vi "Modular Test.vi"() -> ()   [LabVIEW 2018]
uses:
  Classes/Realsense Cam/Private/Stream Config STYP.ctl
  Classes/Realsense Cam/Private/Stream Types Enum STYP.ctl
  Classes/Message/Message.lvclass
  Classes/Video Cam Processor/Video Cam Processor.lvclass
  C:/Users/aaron.jencks/Documents/GitHub/emerson_seed_object_detection/LabVIEW/Projects/Paul's Video Viewer/Classes/Realsense Cam Video File Wrapper/Realsense Cam File Wrapper.lvclass
  C:/Users/aaron.jencks/Documents/GitHub/emerson_seed_object_detection/LabVIEW/Projects/Paul's Video Viewer/Classes/Video Processor/Video Processor.lvclass
  Classes/Frame Data Message/Frame Data Message.lvclass
  C:/Users/aaron.jencks/Documents/GitHub/emerson_seed_object_detection/LabVIEW/Projects/Paul's Video Viewer/Classes/Message/Message.lvclass
  Classes/STOP Message/STOP.lvclass
  Classes/Realsense Cam/Realsense Cam.lvclass
  Classes/Image Processing Handler/Image Processing Handler.lvclass
panel:
  out "Image":T1(plugin-control)
  in  "stop":bool
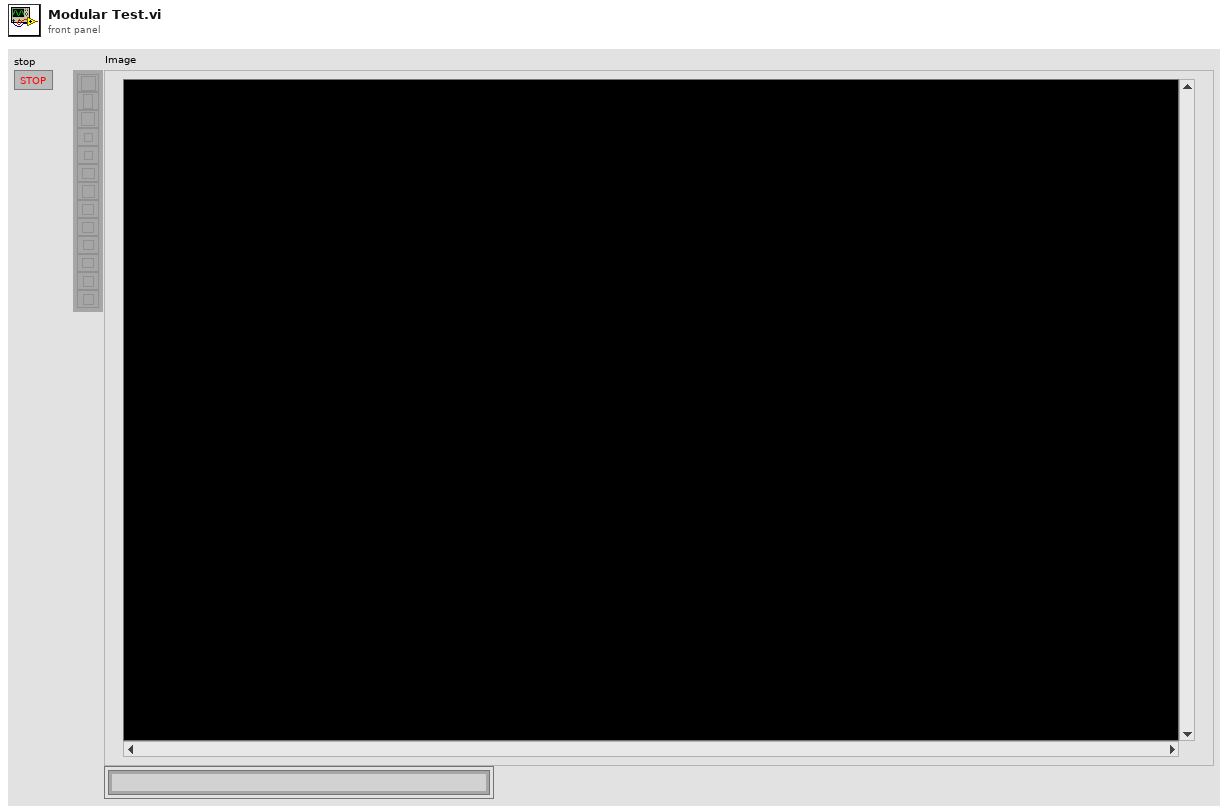
[diagram p1: front panel]
types:
  T1 = typedef "IMAQ Image.ctl" = refnum<image>
  T2 = typedef "Realsense Cam.lvclass/Stream Config STYP.ctl" = cluster{"Stream Type":T3, "Resolution":u16}
  T3 = typedef "Realsense Cam.lvclass/Stream Types Enum STYP.ctl" = enum16{"Depth", "Left IR", "Left IR Unrectified", "Right IR", "Right IR Unrectified", "Color", "RGB Ext."}
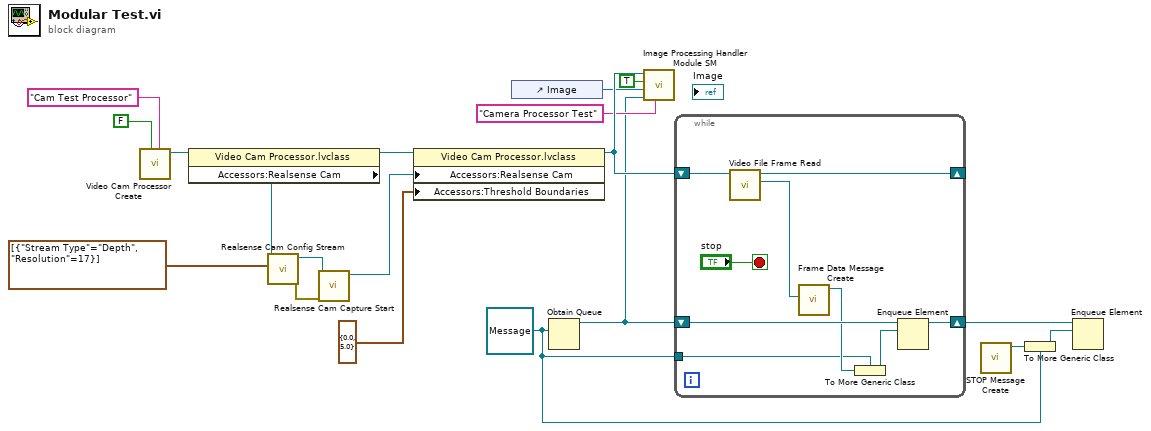
[diagram p0: block diagram]
diagram:
  w2 = refnum<class "Message.lvclass"> refnum ("Message.lvclass")
  n1 = call "Video Cam Processor Create.vi"("Identifier"="Cam Test Processor", "Open? (T)"=FALSE) -> ("Video Processor out"=w16:refnum<class "Video Cam Processor.lvclass">)  [unwired: 8 in, 1 out]
  n2 = property class="Video Cam Processor.lvclass"(reference=w16) -> (reference out=w13:refnum<class "Video Cam Processor.lvclass">, "Accessors:Realsense Cam"=w15:refnum<class "Realsense Cam.lvclass">)  [unwired: 1 in, 1 out]
  n3 = call-dynamic "Realsense Cam Config Stream.vi"("Streams"=T2[] [{"Stream Type"=enum."Depth", "Resolution"=17}], "Realsense Cam in"=w15) -> ("error out"=w17:errorcluster, "Realsense Cam out"=w18:refnum<class "Realsense Cam.lvclass">)  [unwired: 8 in]
  n4 = call-dynamic "Realsense Cam Capture Start.vi"("error in (no error)"=w17, "Realsense Cam in"=w18) -> ("Realsense Cam out"=w12:refnum<class "Realsense Cam.lvclass">)  [unwired: 7 in, 2 out]
  n5 = property class="Video Cam Processor.lvclass"(reference=w13, "Accessors:Realsense Cam"=w12, "Accessors:Threshold Boundaries"=cluster{"Minimum":dbl, "Maximum":dbl} {"Minimum"=0.0, "Maximum"=5.0} ("Threshold Boundaries")) -> (reference out=w9:refnum<class "Video Cam Processor.lvclass">)  [unwired: 1 in, 1 out]
  n6 = control-ref of="Image"() -> (w7:refnum<vi>)
  n7 = Obtain Queue(element data type=w2) -> (queue out=w5:refnum<queue>)  [unwired: 4 in, 2 out]
  n8 = call "Image Processing Handler Module SM.vi"("Identifier"="Camera Processor Test", "data queue"=w5, "Image Ctl Refnum"=w7, "Camera? (F)"=TRUE, "Video Processor"=w9) -> ()  [unwired: 7 in]
  n9 = while {
    shift-right: [w21] -> _
    shift-left: w9 -> [w28]
    tunnel: w2 -> [w23]
    shift-right: [w20] -> w4
    shift-left: w5 -> [w25]
    stop <- "stop" stop-if-true
    n10 = call-dynamic "Video File Frame Read.vi"("Video Processor in"=w28) -> ("Video Frame out"=w26:refnum<class "Video Frame.lvclass">, "Video Processor out"=w21:refnum<class "Video Cam Processor.lvclass">)  [unwired: 6 in, 3 out]
    n11 = call "Frame Data Message Create.vi"("Video Frame"=w26) -> ("Frame Data Message out"=w24:refnum<class "Frame Data Message.lvclass">)  [unwired: 9 in, 1 out]
    n12 = To More Generic Class(target class=w23, reference=w24) -> (generic class reference=w22:refnum<class "Message.lvclass">)
    n13 = Enqueue Element(queue=w25, element=w22) -> (queue out=w20:refnum<queue>)  [unwired: 2 in, 2 out]
  }
  n14 = call "STOP Message Create.vi"() -> ("STOP out"=w3:refnum<class "STOP.lvclass">)  [unwired: 10 in, 1 out]
  n15 = To More Generic Class(target class=w2, reference=w3) -> (generic class reference=w1:refnum<class "Message.lvclass">)
  n16 = Enqueue Element(queue=w4, element=w1) -> ()  [unwired: 2 in, 3 out]
